vi "saveToDatabase.vi"(0 "Connection":string, 1 "Data":variant, 5 "Table":string, 7 "Auto Increment ID?":bool, 9 "Delete row?":bool, 11 "Error in":errorcluster, 12 "Maximum Row":i32, 13 "Delete Method":enum16{"ID Delete", "Time Delete"}(ring)) -> (15 "Error out":errorcluster)   [LabVIEW 2020, in "databaseLibrary.lvlib"]
uses:
  databaseLibrary.lvlib
  <vilib>/addons/database/Connection.llb/DB Tools Open Connec (String).vi
  <vilib>/addons/database/_DB Variant To Data/Database Variant To Data.xnode
  <vilib>/addons/database/NI_Database_API.lvlib
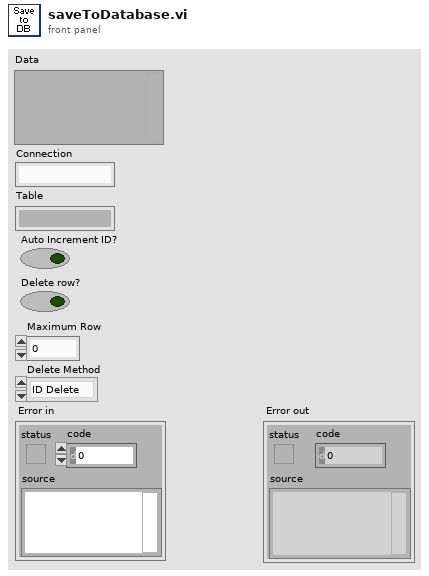
[diagram p1: front panel]
types:
  T1 = typedef "NI_Database_API.lvlib/Conn ObjectReference.ctl" = refnum<k1>
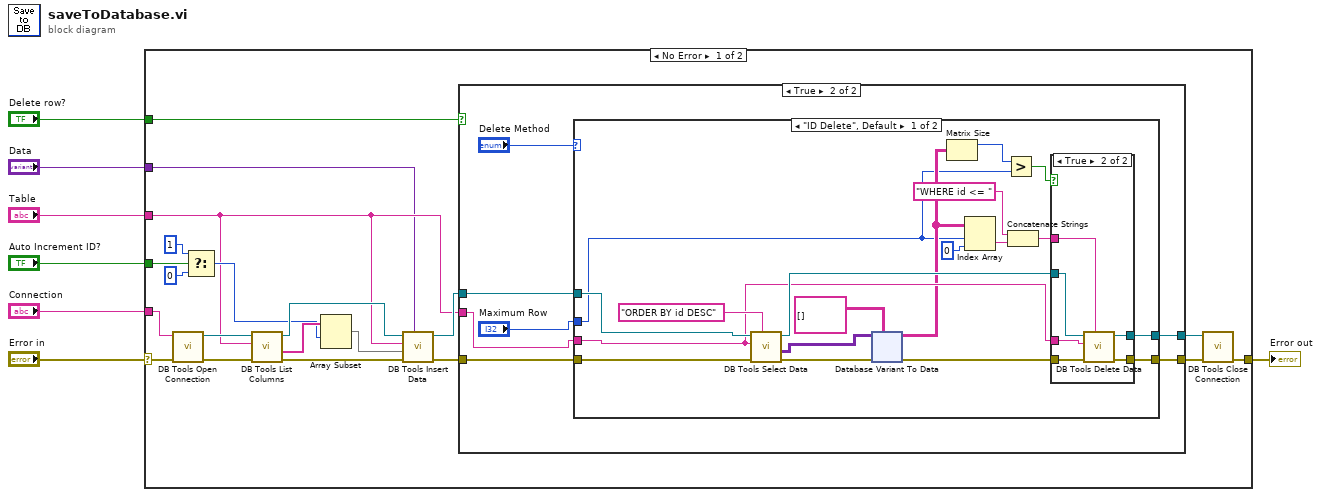
[diagram p0: block diagram]
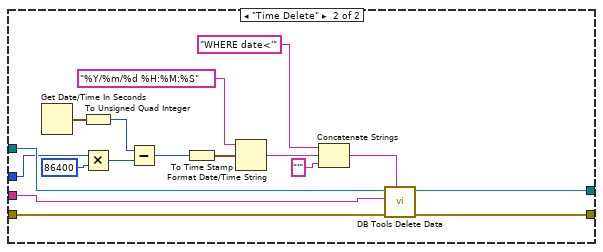
[diagram p4: hidden frame]
diagram:
  n1 = case shown="No Error" "Error in" {
    selector: "Error in" -> [w8 w125]
    tunnel: "Connection" -> [w21 _]
    tunnel: "Auto Increment ID?" -> [w20 _]
    tunnel: "Table" -> [w14 _]
    tunnel: "Data" -> [w13 _]
    tunnel: "Delete row?" -> [w12 _]
    tunnel: [w11 w125] -> w2
    frame No Error {
      n2 = call-poly <vilib>:"DB Tools Open Connection.vi"("error in (no error)"=w8, "connection information"=w21) -> ("error out"=w25:errorcluster, "connection reference"=w27:T1)  [unwired: 6 in]
      n3 = Select(t=1 ("index"), s=w20, f=0) -> (s? t:f=w16:i32)
      n4 = call <vilib>:"DB Tools List Columns.vi"("error in (no error)"=w25, "table"=w14, "connection reference"=w27) -> ("error out"=w24:errorcluster, "columns"=w19:string[], "connection reference out"=w26:T1)  [unwired: 1 in, 1 out]
      n5 = Array Subset(array=w19, index=w16) -> (w15:string[])  [unwired: 1 in]
      n6 = call <vilib>:"DB Tools Insert Data.vi"("data"=w13, "error in (no error)"=w24, "columns"=w15, "table"=w14, "connection reference"=w26) -> ("error out"=w23:errorcluster, "connection reference out"=w22:T1)  [unwired: 5 in]
      n7 = case shown="True" w12 {
        tunnel: w23 -> [w28 w36]
        tunnel: w22 -> [w29 w35]
        tunnel: w14 -> [_ w34]
        tunnel: [w28 w33] -> w10
        tunnel: [w29 w32] -> w9
        frame False {
        }
        frame True {
          n8 = case shown="\"ID Delete\", Default" "Delete Method" {
            tunnel: w36 -> [w54 w124]
            tunnel: w35 -> [w55 w123]
            tunnel: w34 -> [w43 w122]
            tunnel: [w46 w121] -> w33
            tunnel: [w45 w120] -> w32
            tunnel: "Maximum Row" -> [w41 w108]
            frame "ID Delete", Default {
              n9 = call <vilib>:"DB Tools Select Data.vi"("condition"="ORDER BY id DESC", "error in (no error)"=w54, "table"=w43, "connection reference"=w55) -> ("error out"=w52:errorcluster, "data"=w53:variant[][], "connection reference out"=w44:T1)  [unwired: 2 in]
              n10 = xnode "Database Variant To Data"("database variant"=w53, "error in (no error)"=w52, "type"=string[][] []) -> ("data"=w42:string[][], "error out"=w47:errorcluster)
              n11 = Matrix Size(0:w42) -> (1:w49:i32)  [unwired: 1 out]
              n12 = Index Array(array=w42, index (row)=w41, index (col)=0 ("disabled index (col)")) -> (element=w39:string)
              n13 = Greater?(x=w49, y=w41) -> (0:w48:bool)
              n14 = Concatenate Strings("WHERE id <= " ("string"), w39) -> (w37:string)
              n15 = case shown="True" w48 {
                tunnel: w47 -> [w57 w63]
                tunnel: [w57 w62] -> w46
                tunnel: [w56 w61] -> w45
                tunnel: w44 -> [w56 w60]
                tunnel: w43 -> [_ w59]
                tunnel: w37 -> [_ w58]
                frame False {
                }
                frame True {
                  n16 = call <vilib>:"DB Tools Delete Data.vi"("condition"=w58, "error in (no error)"=w63, "table"=w59, "connection reference"=w60) -> ("error out"=w62:errorcluster, "connection reference out"=w61:T1)  [unwired: 6 in]
                }
              }
            }
            frame "Time Delete" {
              n17 = Get Date/Time In Seconds() -> (seconds since 1Jan1904=w115:timestamp)
              n18 = To Unsigned Quad Integer(1:w115) -> (0:w118:u64)
              n19 = Multiply(x=w108, y=u64 86400) -> (x*y=w117:u64)
              n20 = Subtract(x=w118, y=w117) -> (x-y=w119:u64)
              n21 = To Time Stamp(1:w119) -> (0:w114:timestamp)
              n22 = Format Date/Time String(time format string (%c)="%Y/%m/%d %H:%M:%S", seconds (now)=w114) -> (date/time string=w116:string)  [unwired: 1 in]
              n23 = Concatenate Strings("WHERE date<'" ("string"), w116, "'" ("string")) -> (w109:string)
              n24 = call <vilib>:"DB Tools Delete Data.vi"("condition"=w109, "error in (no error)"=w124, "table"=w122, "connection reference"=w123) -> ("error out"=w121:errorcluster, "connection reference out"=w120:T1)  [unwired: 6 in]
            }
          }
        }
      }
      n25 = call <vilib>:"DB Tools Close Connection.vi"("error in (no error)"=w10, "connection reference"=w9) -> ("error out"=w11:errorcluster)  [unwired: 5 in]
    }
    frame Error {
    }
  }
  "Error out" <- w2
